vi "clearReadings.vi"(8 "error in (no error)":errorcluster, 11 "ElectrometerController in":refnum<class "ElectrometerController.lvclass">) -> (0 "error out":errorcluster, 3 "ElectrometerController out":refnum<class "ElectrometerController.lvclass">)   [LabVIEW 2016, in "ElectrometerController.lvclass"]
uses:
  ElectrometerController.lvclass
  ts_electrometeruserevents/Typedefs/Reading.ctl
  ElectrometerController.lvclass/ElectrometerController.ctl
  ts_electrometeruserevents/Typedefs/ElectrometerTypedefs.lvlib
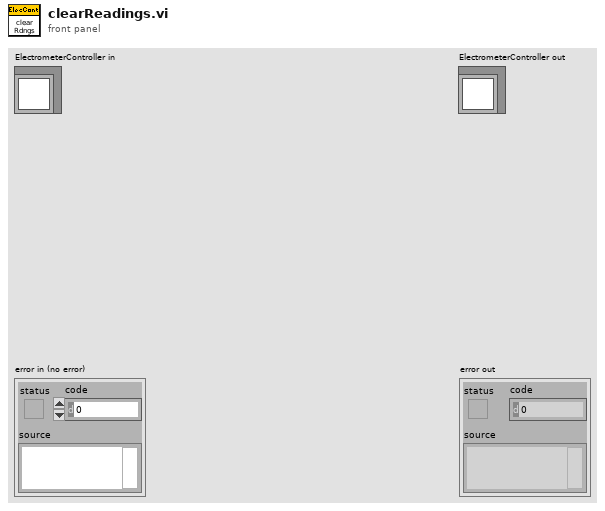
[diagram p1: front panel]
types:
  T1 = typedef "ElectrometerTypedefs.lvlib/Reading.ctl" = cluster{"intensity":dbl, "Unit":string, "temperature":dbl}
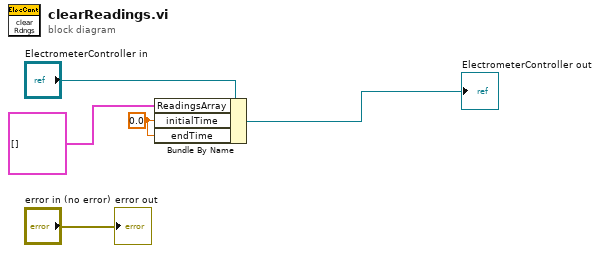
[diagram p0: block diagram]
diagram:
  w1 = 0.0 ("initialTime")
  n1 = Bundle By Name(cluster="ElectrometerController in", "ReadingsArray"=T1[] [], "initialTime"=w1, "endTime"=w1) -> (→"ElectrometerController out":refnum<class "ElectrometerController.lvclass">)
  "error out" <- "error in (no error)"
